vi "AM Modulation Demo (Baseband-Sine) - Basic.vi"() -> ()   [LabVIEW 2013]
uses:
  <vilib>/express/express analysis/Spectral/Block/exnSpectralBlock spectral measurements power poly.vi
  <vilib>/express/express analysis/Spectral/Block/exnSpectralBlock spectral measurements power DDT.vi
  <vilib>/express/express analysis/Spectral/XNode/ExpressSpectralMeasurementsBlockNode.xnode
panel:
  out "After Rectifier 2":dynamicdata(graph)=[{"t0"=timestamp(0 s since 1904-01-01), "dt"=10.0, "Y"=array[50000 elements], "attributes"=variant("NI_ChannelName"=variant(string "Sine (Power Spectrum)"), "NI_ExpIsRelativeTime"=variant(bool TRUE), "NI_ExpStartTimeStamp"=variant(timestamp timestamp(3635665779.2842293 s since 1904-01-01)), "NI_ExpTimeStamp"=variant(timestamp timestamp(3635665779.2842293 s since 1904-01-01)), "NI_ExpXDimension"=variant(string "f"), "NI_OriginalChannelName"=variant(string "Sine"))}]
  in  "WAV Sample Rate":dbl=44100.0 caption="dt"
  in  "Mod Freq.":dbl=2000.0 caption="Frequency"
  in  "LPF Cut-Off":dbl=10000.0 caption="Lower Cut-Off"
  in  "AWGN (dB)":dbl(slide)=0.6 caption="Standard deviation" scale=-20.0..50.0
  out "Comparision":dynamicdata(graph)
  out "Baseband":dynamicdata(graph)
  out "AM Power Spectrum":dynamicdata(graph)
  out "AM Wave":dynamicdata(graph)
  in  "DC Offset":dbl=1.0
  in  "Carrier Amp.":dbl=1.0 caption="Amplitude"
  in  "stop":bool
  in  "Modulation Index":dbl(slide)=1.0 scale=0.0..5.0
  in  "Carrier Freq.":dbl=100000.0 caption="Frequency"
  out "After Rectifier":dynamicdata(graph)=[{"t0"=timestamp(0 s since 1904-01-01), "dt"=10.0, "Y"=array[50000 elements], "attributes"=variant("NI_ChannelName"=variant(string "Sine (Power Spectrum)"), "NI_ExpIsRelativeTime"=variant(bool TRUE), "NI_ExpStartTimeStamp"=variant(timestamp timestamp(3635665779.2842293 s since 1904-01-01)), "NI_ExpTimeStamp"=variant(timestamp timestamp(3635665779.2842293 s since 1904-01-01)), "NI_ExpXDimension"=variant(string "f"), "NI_OriginalChannelName"=variant(string "Sine"))}]
  # "Amplitude Modulation"
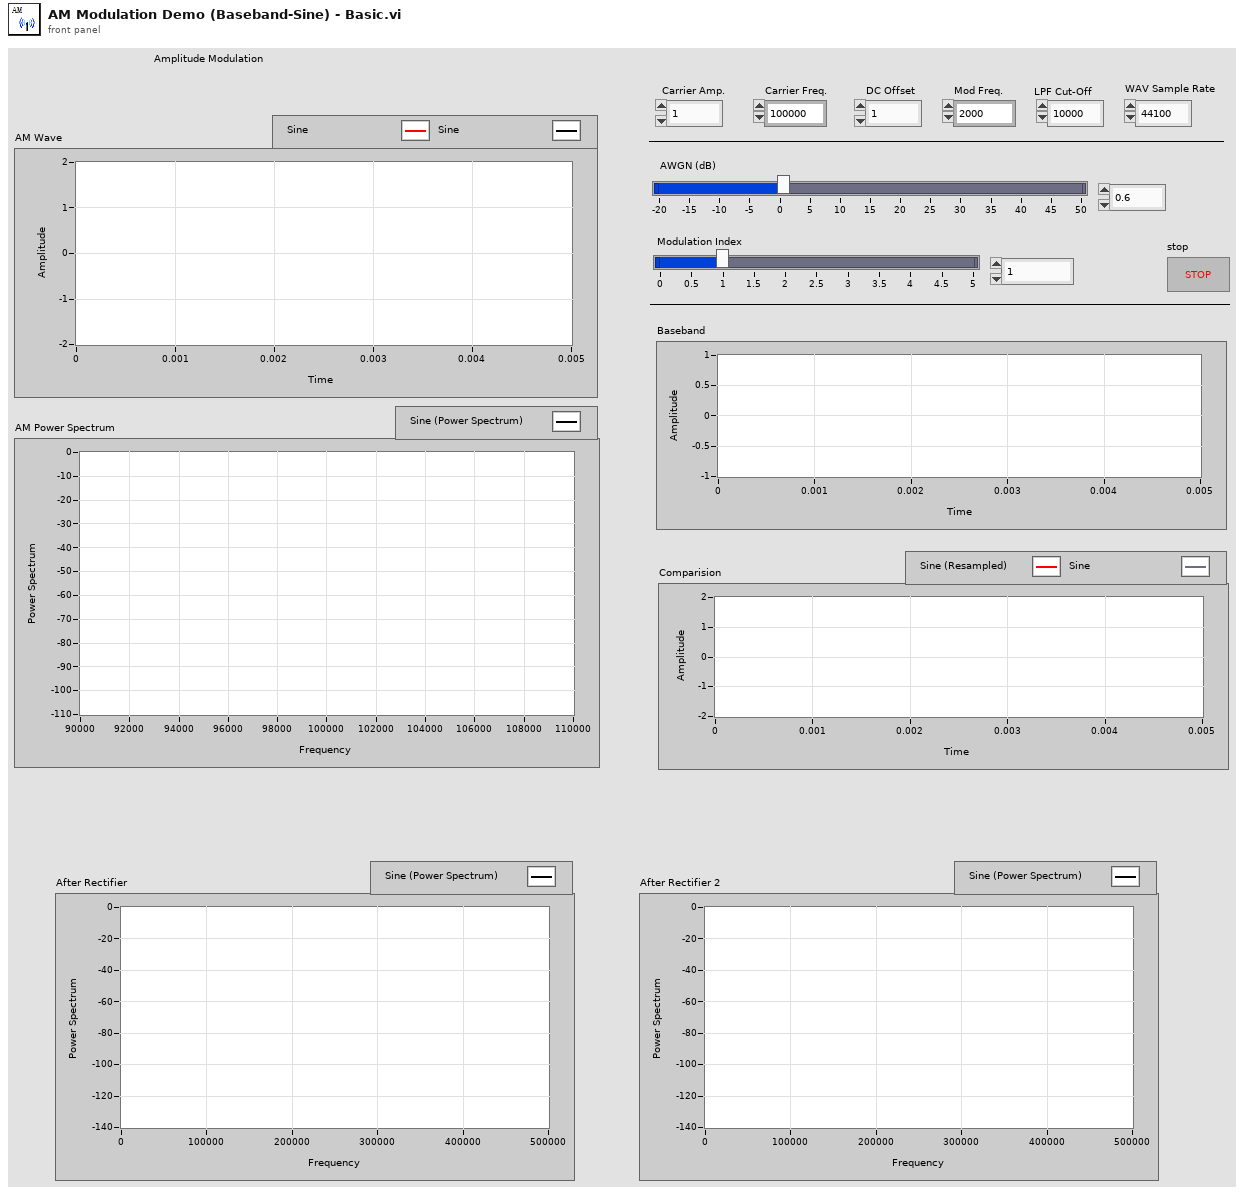
[diagram p1: front panel]
types:
  T1 = cluster{"averaging mode":u16, "weighting mode":u16, "number of averages":u32}
  T2 = cluster{"dB On (F)":bool, "unwrap phase (F)":bool, "convert to degree (F)":bool}
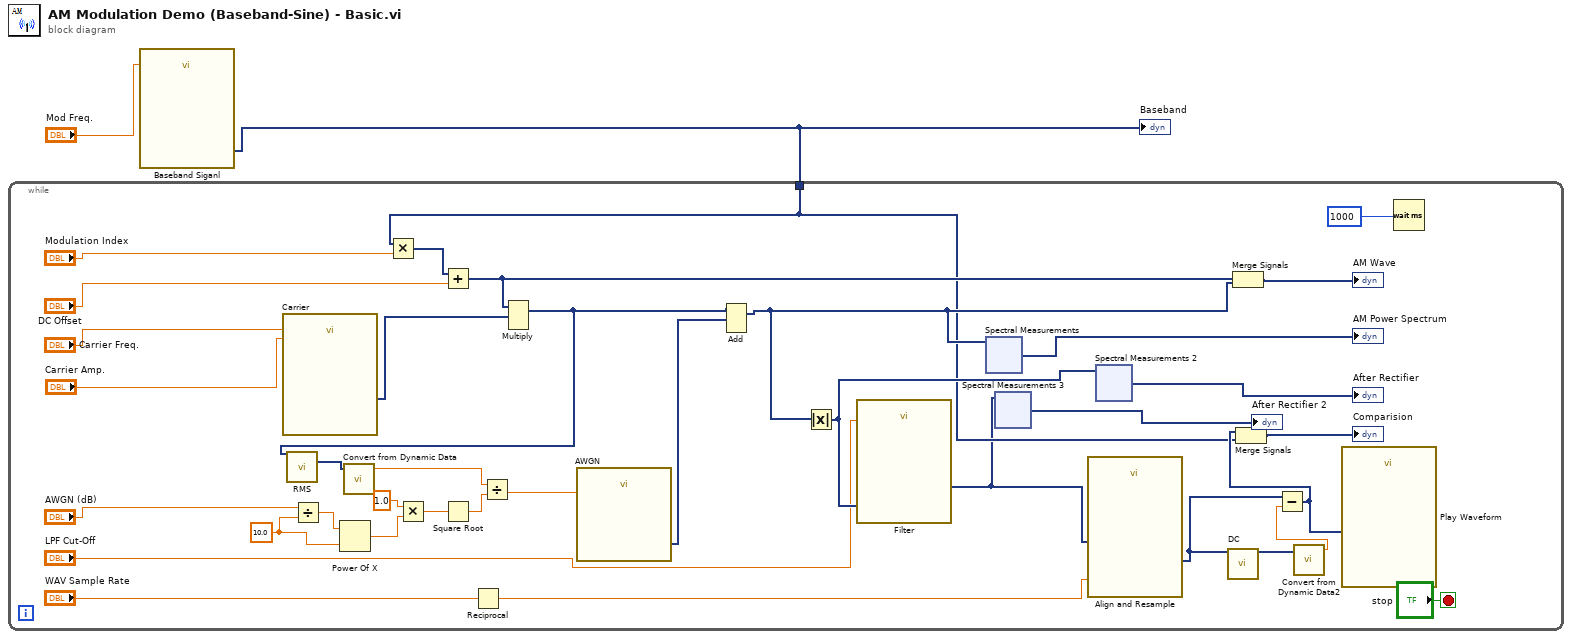
[diagram p0: block diagram]
diagram:
  n1 = call "Baseband Siganl"("Frequency"="Mod Freq.") -> ("Sine"=w1:dynamicdata)  [unwired: 13 in, 1 out]
  "Baseband" <- w1
  n2 = while {
    tunnel: w1 -> [w7]
    stop <- "stop" stop-if-true
    w21 = 10.0
    n3 = call "Carrier"("Frequency"="Carrier Freq.", "Amplitude"="Carrier Amp.") -> ("Sine"=w30:dynamicdata)  [unwired: 12 in, 1 out]
    n4 = Divide(x="AWGN (dB)", y=w21) -> (x/y=w27:dbl)
    n5 = Power Of X(1:w21, 2:w27) -> (0:w25:dbl)
    n6 = Multiply(x=w7, y="Modulation Index") -> (x*y=w37:dynamicdata)
    n7 = Multiply(x=1.0, y=w25) -> (x*y=w24:dbl)
    n8 = Add(x=w37, y="DC Offset") -> (x+y=w33:dynamicdata)
    n9 = Square Root(x=w24) -> (sqrt(x)=w23:dbl)
    n10 = Reciprocal(x="WAV Sample Rate") -> (1/x=w9:dbl)
    n11 = Multiply(1:w30, 2:w33) -> (0:w20:dynamicdata)  [unwired: 1 in, 1 out]
    n12 = call "RMS"("Signals"=w20) -> ("RMS"=w3:dynamicdata)  [unwired: 13 in, 1 out]
    n13 = call "Convert from Dynamic Data"("Dynamic Data Type"=w3) -> ("Scalar"=w22:dbl)  [unwired: 3 in]
    n14 = Divide(x=w22, y=w23) -> (x/y=w18:dbl)
    n15 = call "AWGN"("Standard deviation"=w18) -> ("DC with Gaussian Noise"=w19:dynamicdata)  [unwired: 13 in, 1 out]
    n16 = Add(1:w19, 2:w20) -> (0:w17:dynamicdata)  [unwired: 1 in, 1 out]
    n17 = Absolute Value(x=w17) -> (abs(x)=w16:dynamicdata)
    n18 = call "Filter"("Lower Cut-Off"="LPF Cut-Off", "Signal"=w16) -> ("Filtered Signal"=w4:dynamicdata)  [unwired: 8 in, 1 out]
    n19 = xnode "Spectral Measurements"("Signals"=w17) -> ("Power Spectrum"=→"AM Power Spectrum":dynamicdata)  [unwired: 1 in, 1 out]
    n20 = xnode "Spectral Measurements 3"("Signals"=w4) -> ("Power Spectrum"=→"After Rectifier 2":dynamicdata)  [unwired: 1 in, 1 out]
    n21 = call "Align and Resample"("dt"=w9, "Signals"=w4) -> ("Resampled Signals"=w13:dynamicdata)  [unwired: 7 in, 2 out]
    n22 = xnode "Spectral Measurements 2"("Signals"=w16) -> ("Power Spectrum"=→"After Rectifier":dynamicdata)  [unwired: 1 in, 1 out]
    n23 = call "DC"("Signals"=w13) -> ("Mean (DC)"=w11:dynamicdata)  [unwired: 13 in, 1 out]
    n24 = Merge Signals(w33, w17) -> (→"AM Wave":dynamicdata)
    n25 = call "Convert from Dynamic Data2"("Dynamic Data Type"=w11) -> ("Scalar"=w12:dbl)  [unwired: 3 in]
    n26 = Subtract(x=w13, y=w12) -> (x-y=w8:dynamicdata)
    n27 = Merge Signals(w8, w7) -> (→"Comparision":dynamicdata)
    n28 = call "Play Waveform"("Data"=w8) -> ()  [unwired: 18 in, 1 out]
    n29 = Wait (ms)(milliseconds to wait=1000) -> ()  [unwired: 1 out]
  }
